vi "Compute Trigger Signal.vi"(2 "IBP Out":cluster{"IBP1":i16, "IBP2":i16}, 3 "Filtered Leads":T1, 4 "Trigger":T2) -> (0 "Trigger Out":bool, 1 "Leads Out":T1)   [LabVIEW 2016]
uses:
  ECG Leads.ctl
  Trigger Params.ctl
  Channel Enum.ctl
  <vilib>/rvi/Analysis/measure/butterworth/XNode/niFpgaButterworthFilter.xnode
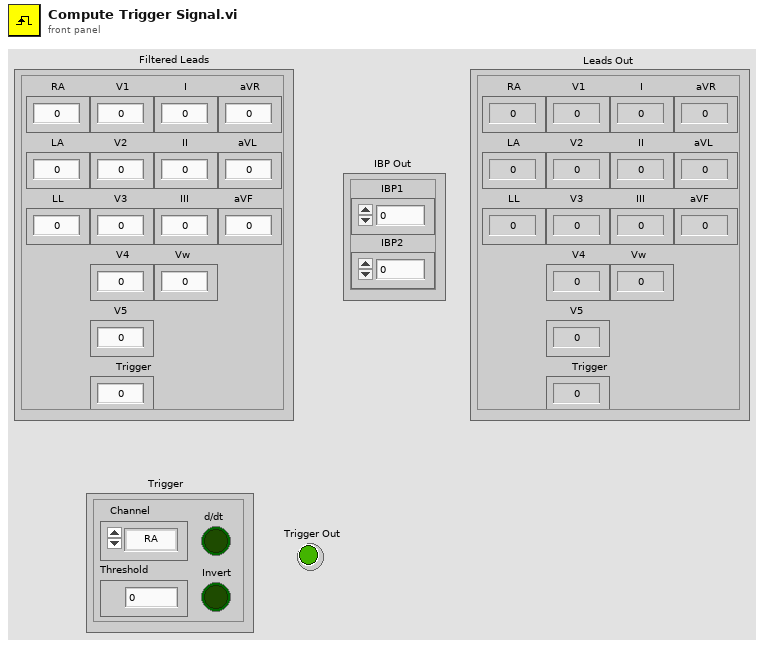
[diagram p1: front panel]
types:
  T1 = typedef "ECG Leads.ctl" = cluster{"RA":i16, "LA":i16, "LL":i16, "V1":i16, "V2":i16, "V3":i16, "V4":i16, "V5":i16, "Trigger":i16, "I":i16, "II":i16, "III":i16, "aVR":i16, "aVL":i16, "aVF":i16, "Vw":i16}
  T2 = typedef "Trigger Params.ctl" = cluster{"Channel":T3, "Threshold":i16, "d/dt":bool, "Invert":bool}
  T3 = typedef "Channel Enum.ctl" = enum16{"RA", "LA", "LL", "V1", "V2", "V3", "V4", "V5", "V6", "I", "II", "III", "aVR", "aVL", "aVF", "Vw", "IBP1", "IBP2"}
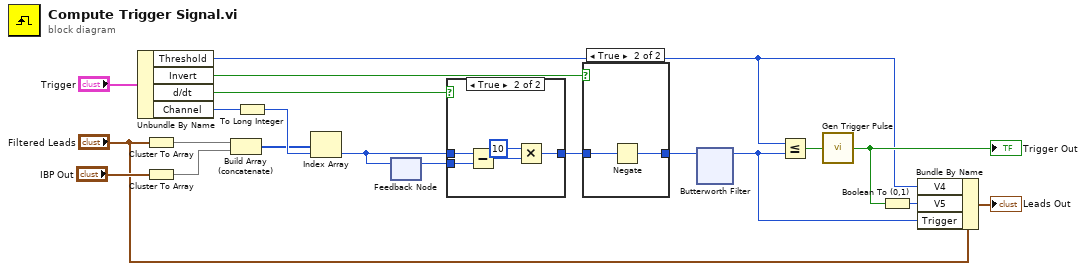
[diagram p0: block diagram]
diagram:
  n1 = Unbundle By Name("Trigger") -> ("Threshold"=w2:i16, "Invert"=w10:bool, "d/dt"=w11:bool, "Channel"=w18:T3)
  n2 = Cluster To Array(cluster="Filtered Leads") -> (array=w19:i16[])
  n3 = Cluster To Array(cluster="IBP Out") -> (array=w14:i16[])
  n4 = Build Array (concatenate)(w19, w14) -> (w15:i16[])
  n5 = To Long Integer(number=w18) -> (32bit integer=w17:i32)
  n6 = Index Array(array=w15, index=w17) -> (element=w1:i16)
  n7 = feedback-in #1(w1) -> ()
  n8 = feedback #1() -> (w13:i16)  [unwired: 1 in]
  n9 = case shown="True" w11 {
    tunnel: w1 -> [w21 w24]
    tunnel: w13 -> [_ w26]
    tunnel: [w21 w23] -> w12
    frame False {
    }
    frame True {
      n10 = Subtract(x=w24, y=w26) -> (x-y=w25:i16)
      n11 = Multiply(x=i16 10, y=w25) -> (x*y=w23:i16)
    }
  }
  n12 = case shown="True" w10 {
    tunnel: w12 -> [w27 w29]
    tunnel: [w27 w28] -> w7
    frame False {
    }
    frame True {
      n13 = Negate(x=w29) -> (-x=w28:i16)
    }
  }
  n14 = xnode "Butterworth Filter"("input data"=w7) -> ("output data"=w6:i16)  [unwired: 2 in]
  n15 = Less Or Equal?(x=w2, y=w6) -> (x <= y?=w5:bool)
  n16 = call "Gen Trigger Pulse.vi"("Threshold In"=w5) -> ("Threshold Out"=w3:bool)  [unwired: 2 in]
  "Trigger Out" <- w3
  n17 = Boolean To (0,1)(Boolean=w3) -> (0, 1=w4:i16)
  n18 = Bundle By Name(cluster="Filtered Leads", "V4"=w2, "V5"=w4, "Trigger"=w6) -> (→"Leads Out":T1)
